vi "Frames per axquisition file.vi"(4 "Output frame width":i16, 6 "Output frame height":i16, 7 "Pixel depth":u32(ring) items=["8 bits", "16 bits", "Float", "Complex", "RGB", "HSL"]) -> (0 "Frames per acquisition file":i32, 2 "Image size (pixels)":dbl)   [LabVIEW 2016]
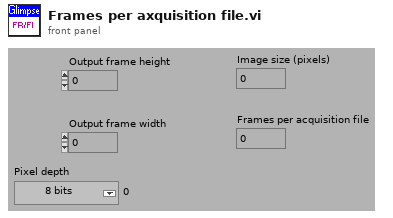
[diagram p1: front panel]
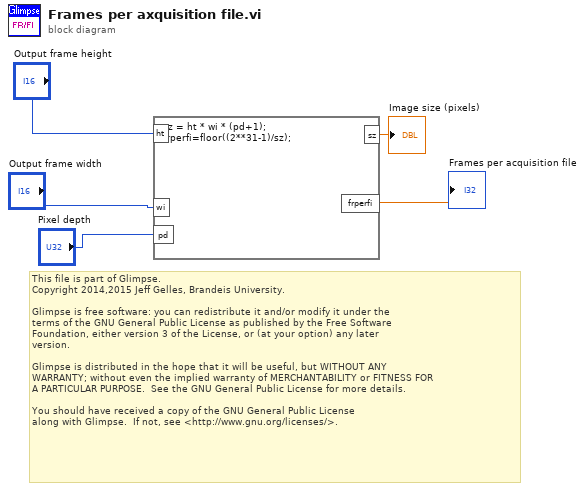
[diagram p0: block diagram]
diagram:
  # "This file is part of Glimpse. \nCopyright 2014,2015 Jeff Gelles, Brandeis University.    \n\nGlimpse is free software: you can redistribute it and/or modify it under the \nterms of the GNU General Public License as published by the Free Software \nFoundation, either version 3 of the License, or (at your option) any later \nversion.\n\nGlimpse is distributed in the hope that it will be useful, but WITHOUT ANY \nWARRANTY; without even the implied warranty of MERCHANTABILITY or FITNESS FOR \nA PARTICULAR PURPOSE.  See the GNU General Public License for more details.\n\nYou should have received a copy of the GNU General Public License\nalong with Glimpse.  If not, see <http://www.gnu.org/licenses/>."
  n1 = formula code="sz = ht * wi * (pd+1);\nfrperfi=floor((2**31-1)/sz);"("ht"="Output frame height", "wi"="Output frame width", "pd"="Pixel depth") -> ("frperfi"=→"Frames per acquisition file":dbl, "sz"=→"Image size (pixels)":dbl)
